vi "From JSON.vi"(8 "error in (no error)":errorcluster, 10 "JSON":string, 11 "Type in":refnum<class "Abs_Value_1D.lvclass">) -> (0 "error out":errorcluster, 3 "Type out":refnum<class "Abs_Value_1D.lvclass">)   [LabVIEW 2021, in "Abs_Value_1D.lvclass"]
uses:
  Abs_Value_1D.lvclass
  Abs_Value_1D.lvclass/Abs_Value_1D.ctl
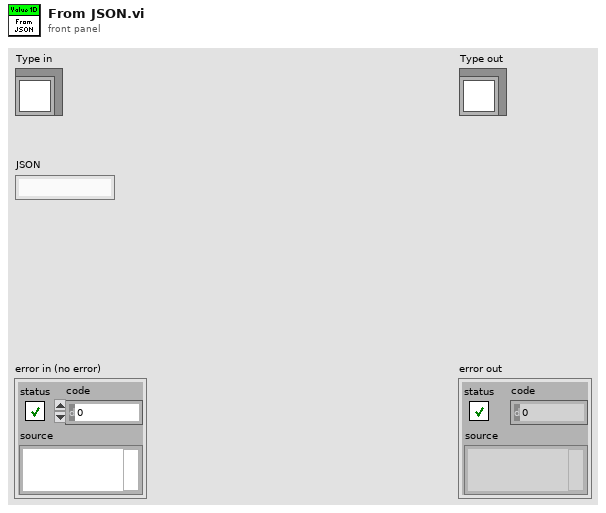
[diagram p1: front panel]
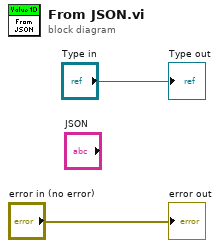
[diagram p0: block diagram]
diagram:
  "error out" <- "error in (no error)"
  "Type out" <- "Type in"
